vi "ADQ214 Set Gain And Offset.vi"(6 "Offset":i32, 7 "Gain":i32, 8 "error in (no error)":errorcluster, 9 "channel":u8, 10 "adq212_num":i32, 11 "adq_cu_ptr":u32) -> (0 "error out":errorcluster, 2 "function return":u32, 3 "adq_cu_ptr out":u32)   [LabVIEW 2013]
doc: "extern \"C\" __declspec(dllimport) unsigned int ADQ214_SetGainAndOffset(void* adq_cu_ptr, int adq212_num, unsigned char channel, int Gain, int Offset);"
uses:
  dlls/ADQAPI.dll
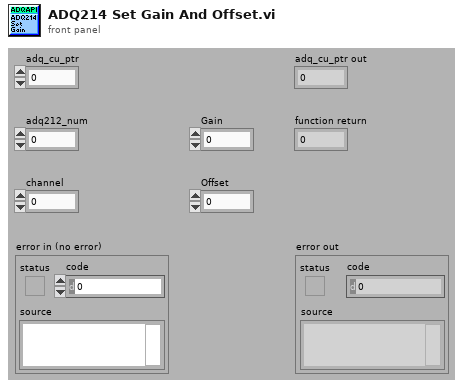
[diagram p1: front panel]
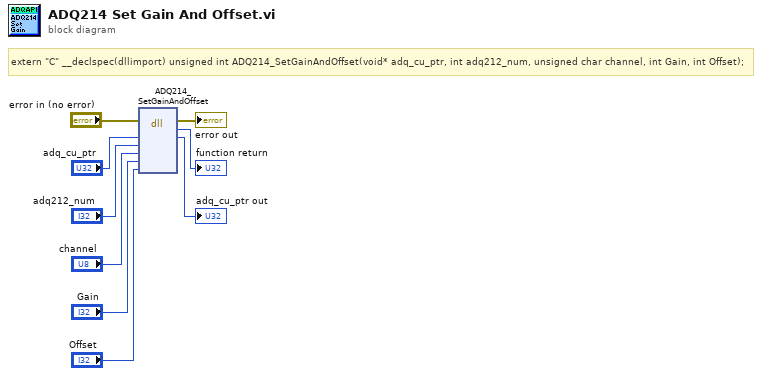
[diagram p0: block diagram]
diagram:
  # "extern \"C\" __declspec(dllimport) unsigned int\tADQ214_SetGainAndOffset(void* adq_cu_ptr, int adq212_num, unsigned char channel, int Gain, int Offset);"
  n1 = dll-call lib="C:/Users/astafiev/Desktop/IlyaDrive/@photonCounting/LabView_Imperium/dlls/ADQAPI.*" fn="ADQ214_SetGainAndOffset"(error in="error in (no error)", "adq_cu_ptr"="adq_cu_ptr", "adq212_num"="adq212_num", "channel"="channel", "Gain"="Gain", "Offset"="Offset") -> (error out=→"error out":errorcluster, "return type"=→"function return":u32, "adq_cu_ptr"=→"adq_cu_ptr out":u32)  [unwired: 6 in, 1 out]
